vi "PKG_IMC_SetPWMfreq.vi"(9 "ch":i32, 10 "freq":dbl, 11 "handle":u32) -> (2 "function return":i32, 3 "handle out":u32)   [LabVIEW 2011, in "IMC_Pkg4xxx.lvlib"]
doc: "PKG_IMC_SetPWMfreq(IMC_HANDLE handle, double freq, int ch);"
uses:
  IMC_Pkg4xxx.lvlib
  IMC_Pkg4xxx.dll
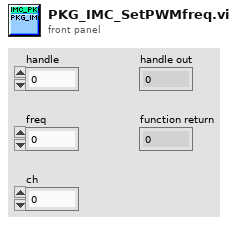
[diagram p1: front panel]
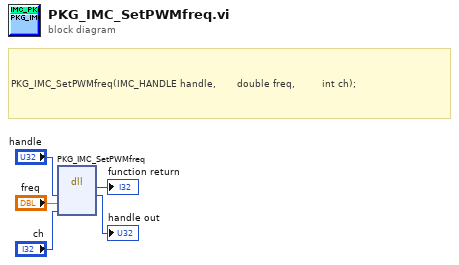
[diagram p0: block diagram]
diagram:
  # "PKG_IMC_SetPWMfreq(IMC_HANDLE handle, \t\t\t\t\t\tdouble freq, \t\t\t\t\t\t\t\tint ch);"
  n1 = dll-call lib="PTH1mabs F光盘刻录\niMC MotionIMCNet_V4.0IMCAppincLabviewIMC_PKG4xxxIMC_PKG4xxx\nIMC_Pkg4xxx.*" fn="PKG_IMC_SetPWMfreq"("handle"="handle", "freq"="freq", "ch"="ch") -> (→"function return":i32, "handle"=→"handle out":u32)  [unwired: 5 in, 2 out]
